vi "openCommunication.vi"(8 "error in (no error)":errorcluster, 11 "Arduino in":refnum<class "Arduino.lvclass">) -> (0 "error out":errorcluster, 3 "Arduino out":refnum<class "Arduino.lvclass">)   [LabVIEW 2020, in "Arduino.lvclass"]
uses:
  Arduino.lvclass
  Arduino.lvclass/Arduino.ctl
  Arduino Shield/Arduino Shield.lvclass
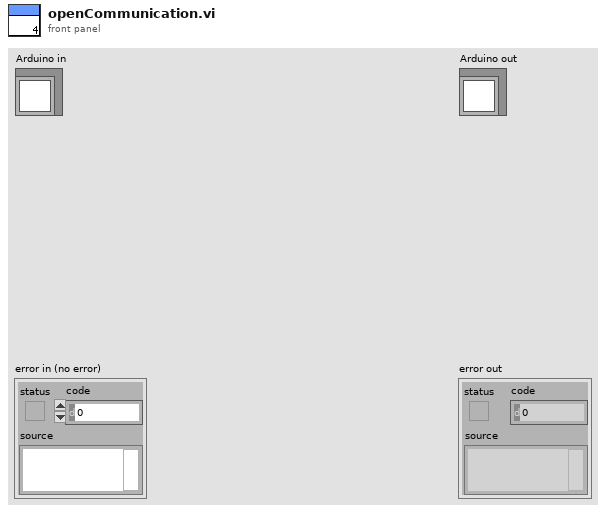
[diagram p1: front panel]
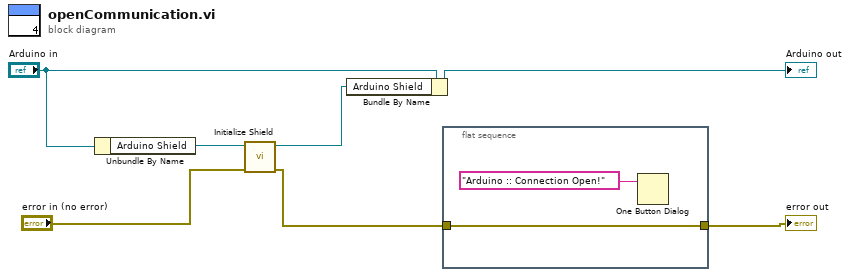
[diagram p0: block diagram]
diagram:
  n1 = Unbundle By Name("Arduino in") -> ("Arduino Shield"=w6:refnum<class "Arduino Shield.lvclass">)
  n2 = call-dynamic "Initialize Shield.vi"("error in (no error)"="error in (no error)", "Arduino Shield in"=w6) -> ("error out"=w2:errorcluster, "Arduino Shield out"=w3:refnum<class "Arduino Shield.lvclass">)  [unwired: 8 in]
  n3 = Bundle By Name(cluster="Arduino in", "Arduino Shield"=w3) -> (→"Arduino out":refnum<class "Arduino.lvclass">)
  n4 = flat-sequence {
    tunnel: w2 -> [w8]
    tunnel: [w8] -> w1
    frame #0 {
      n5 = One Button Dialog(message="Arduino :: Connection Open!") -> ()  [unwired: 1 in, 1 out]
    }
  }
  "error out" <- w1
